vi "WSVCAP SHL Host LL I2C Debug Global.vi"() -> ()   [LabVIEW 2012]
uses:
  Type Defs/WSVCAP SHL Top Level Write Read State Enum.ctl
panel:
  in  "Write Read State":T1
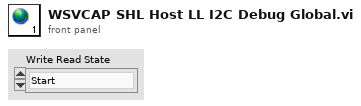
[diagram p1: front panel]
types:
  T1 = typedef "WSVCAP SHL Top Level Write Read State Enum.ctl" = enum16{"Start", "Write", "Read", "Get Status", "Wait Until Done"}
diagram:
